vi "pathplan_vertices_send - 副本 (2).vi"(1 "vertices":dbl[][](array[numeric]), 2 "distance_all":dbl, 3 "angle_all":dbl[](array[numeric]), 4 "speed_max":dbl, 5 "写入串口":refnum<visa-resource-name>) -> (20 "路径规划数据写入缓冲区":string)   [LabVIEW 2016]
uses:
  <vilib>/imath/engines/lvmath2/RunTimeEngine/NodeEndStatement/NIMS_NodeEndStatement_Output.vi
  <instcachedir>/0/NIMS_NodeEndStatement_Output_53EC0D466D134D7ABD903AC30B43404B.lvgen/NIMS_NodeEndStatement_Output_53EC0D466D134D7ABD903AC30B43404B_011.vi
  <instcachedir>/0/NIMS_NodeEndStatement_Output_53EC0D466D134D7ABD903AC30B43404B.lvgen/NIMS_NodeEndStatement_Output_53EC0D466D134D7ABD903AC30B43404B_015.vi
  <vilib>/imath/engines/lvmath2/RunTimeEngine/ErrorHandling/NIMS_Finalize Error.vi
  <vilib>/imath/engines/lvmath2/RunTimeEngine/IndexRead/NIMS M($,S).vi
  <instcachedir>/0/NIMS M($,S)_3E5749BBB62E49528D4765A77F1F6D98.lvgen/NIMS M($,S)_3E5749BBB62E49528D4765A77F1F6D98_000.vi
  <vilib>/imath/engines/lvmath2/RunTimeEngine/ArithmeticOperatorToken/NIMS_ArithmeticOperator_minus.vi
  <instcachedir>/0/NIMS_ArithmeticOperator_minus_E3B65B1D26A44BB184AFDC5B3F458E3D.lvgen/NIMS_ArithmeticOperator_minus_E3B65B1D26A44BB184AFDC5B3F458E3D_003.vi
  <vilib>/imath/engines/lvmath2/RunTimeEngine/BuiltInFunctions/norm/NIMS_norm(GV,DBL).vi
  <instcachedir>/0/NIMS_norm(GV,DBL)_1268AFF3C646412B8C6EA3CE75D09042.lvgen/NIMS_norm(GV,DBL)_1268AFF3C646412B8C6EA3CE75D09042_000.vi
  <vilib>/imath/engines/lvmath2/RunTimeEngine/ErrorHandling/NIMS_Create Error From Enums.vi
  <vilib>/imath/engines/lvmath2/RunTimeEngine/BuiltInFunctions/length/NIMS_length(GM).vi
  <instcachedir>/0/NIMS_length(GM)_47CEC356FCE0482D9BA47DC61C99F2C7.lvgen/NIMS_length(GM)_47CEC356FCE0482D9BA47DC61C99F2C7_000.vi
  <vilib>/imath/engines/lvmath2/RunTimeEngine/RowToken/NIMS_RowToken_M_CV.vi
  <instcachedir>/0/NIMS_RowToken_M_CV_FA79F1D1D17D44459F3ED8E09EE8B625.lvgen/NIMS_RowToken_M_CV_FA79F1D1D17D44459F3ED8E09EE8B625_000.vi
  <vilib>/imathl/engines/lvmath/Functions/Error Handling/Create Error.vi
  <vilib>/imath/engines/lvmath2/RunTimeEngine/IndexRead/NIMS M($,R2).vi
  <instcachedir>/0/NIMS M($,R2)_D9380E19261A4ADFB2D364AF6959C6EF.lvgen/NIMS M($,R2)_D9380E19261A4ADFB2D364AF6959C6EF_001.vi
  <vilib>/imath/engines/lvmath2/RunTimeEngine/BuiltInFunctions/size/NIMS_I32=size(GM,I32).vi
  <instcachedir>/0/NIMS_I32=size(GM,I32)_122058B1B3294FAEA5DC209B92B394E4.lvgen/NIMS_I32=size(GM,I32)_122058B1B3294FAEA5DC209B92B394E4_004.vi
  <vilib>/imath/engines/lvmath2/RunTimeEngine/RangeToken/NIMS_Range_R2 - Integer.vi
  <instcachedir>/0/NIMS_Range_R2 - Integer_89B873E74E6E489885E44F751DD9C6BF.lvgen/NIMS_Range_R2 - Integer_89B873E74E6E489885E44F751DD9C6BF_000.vi
  <vilib>/imath/engines/lvmath2/RunTimeEngine/CommandStatement/MC_CommandStatement_break.vi
  <vilib>/imath/engines/lvmath2/RunTimeEngine/VariableToken/NIMS_VariableToken_CondDefined.vi
  <instcachedir>/0/NIMS_VariableToken_CondDefined_06E9DA95BD4D46A6BA55EC651A891960.lvgen/NIMS_VariableToken_CondDefined_06E9DA95BD4D46A6BA55EC651A891960_009.vi
  <vilib>/imath/engines/lvmath/Functions/Error Handling/MergeErrorsWrapper.vi
  <instcachedir>/0/NIMS_NodeEndStatement_Output_53EC0D466D134D7ABD903AC30B43404B.lvgen/NIMS_NodeEndStatement_Output_53EC0D466D134D7ABD903AC30B43404B_010.vi
  <instcachedir>/0/NIMS_NodeEndStatement_Output_53EC0D466D134D7ABD903AC30B43404B.lvgen/NIMS_NodeEndStatement_Output_53EC0D466D134D7ABD903AC30B43404B_005.vi
  <vilib>/imath/engines/lvmath2/RunTimeEngine/BuiltInFunctions/length/NIMS_length(GV).vi
  <instcachedir>/0/NIMS_length(GV)_08A3D13377FD4E4B96F5795FBF3698FA.lvgen/NIMS_length(GV)_08A3D13377FD4E4B96F5795FBF3698FA_000.vi
  <vilib>/imath/engines/lvmath2/RunTimeEngine/IndexRead/NIMS M(S,S).vi
  <instcachedir>/0/NIMS M(S,S)_AC51E74150A542F7991B9634C66F3096.lvgen/NIMS M(S,S)_AC51E74150A542F7991B9634C66F3096_000.vi
  <vilib>/imath/engines/lvmath2/RunTimeEngine/BuiltInFunctions/dot/NIMS_dot(GV,GV).vi
  <instcachedir>/0/NIMS_dot(GV,GV)_B9FAA411F4494E9B94D442721014A3FA.lvgen/NIMS_dot(GV,GV)_B9FAA411F4494E9B94D442721014A3FA_000.vi
  <vilib>/imath/engines/lvmath2/RunTimeEngine/IndexRead/NIMS V(S).vi
  <instcachedir>/0/NIMS V(S)_0488751826AF41519A22953C041130DC.lvgen/NIMS V(S)_0488751826AF41519A22953C041130DC_000.vi
  <instcachedir>/0/NIMS_NodeEndStatement_Output_53EC0D466D134D7ABD903AC30B43404B.lvgen/NIMS_NodeEndStatement_Output_53EC0D466D134D7ABD903AC30B43404B_009.vi
panel:
  in  "y":dbl
  in  "x":dbl
  in  "angle_z":sgl
  out "vertices_set":i32[][](array[numeric])
  out "angle_send":dbl[](array[numeric])
  out "vertices_send":dbl[](array[numeric])
  out "speed_send":dbl[](array[numeric])
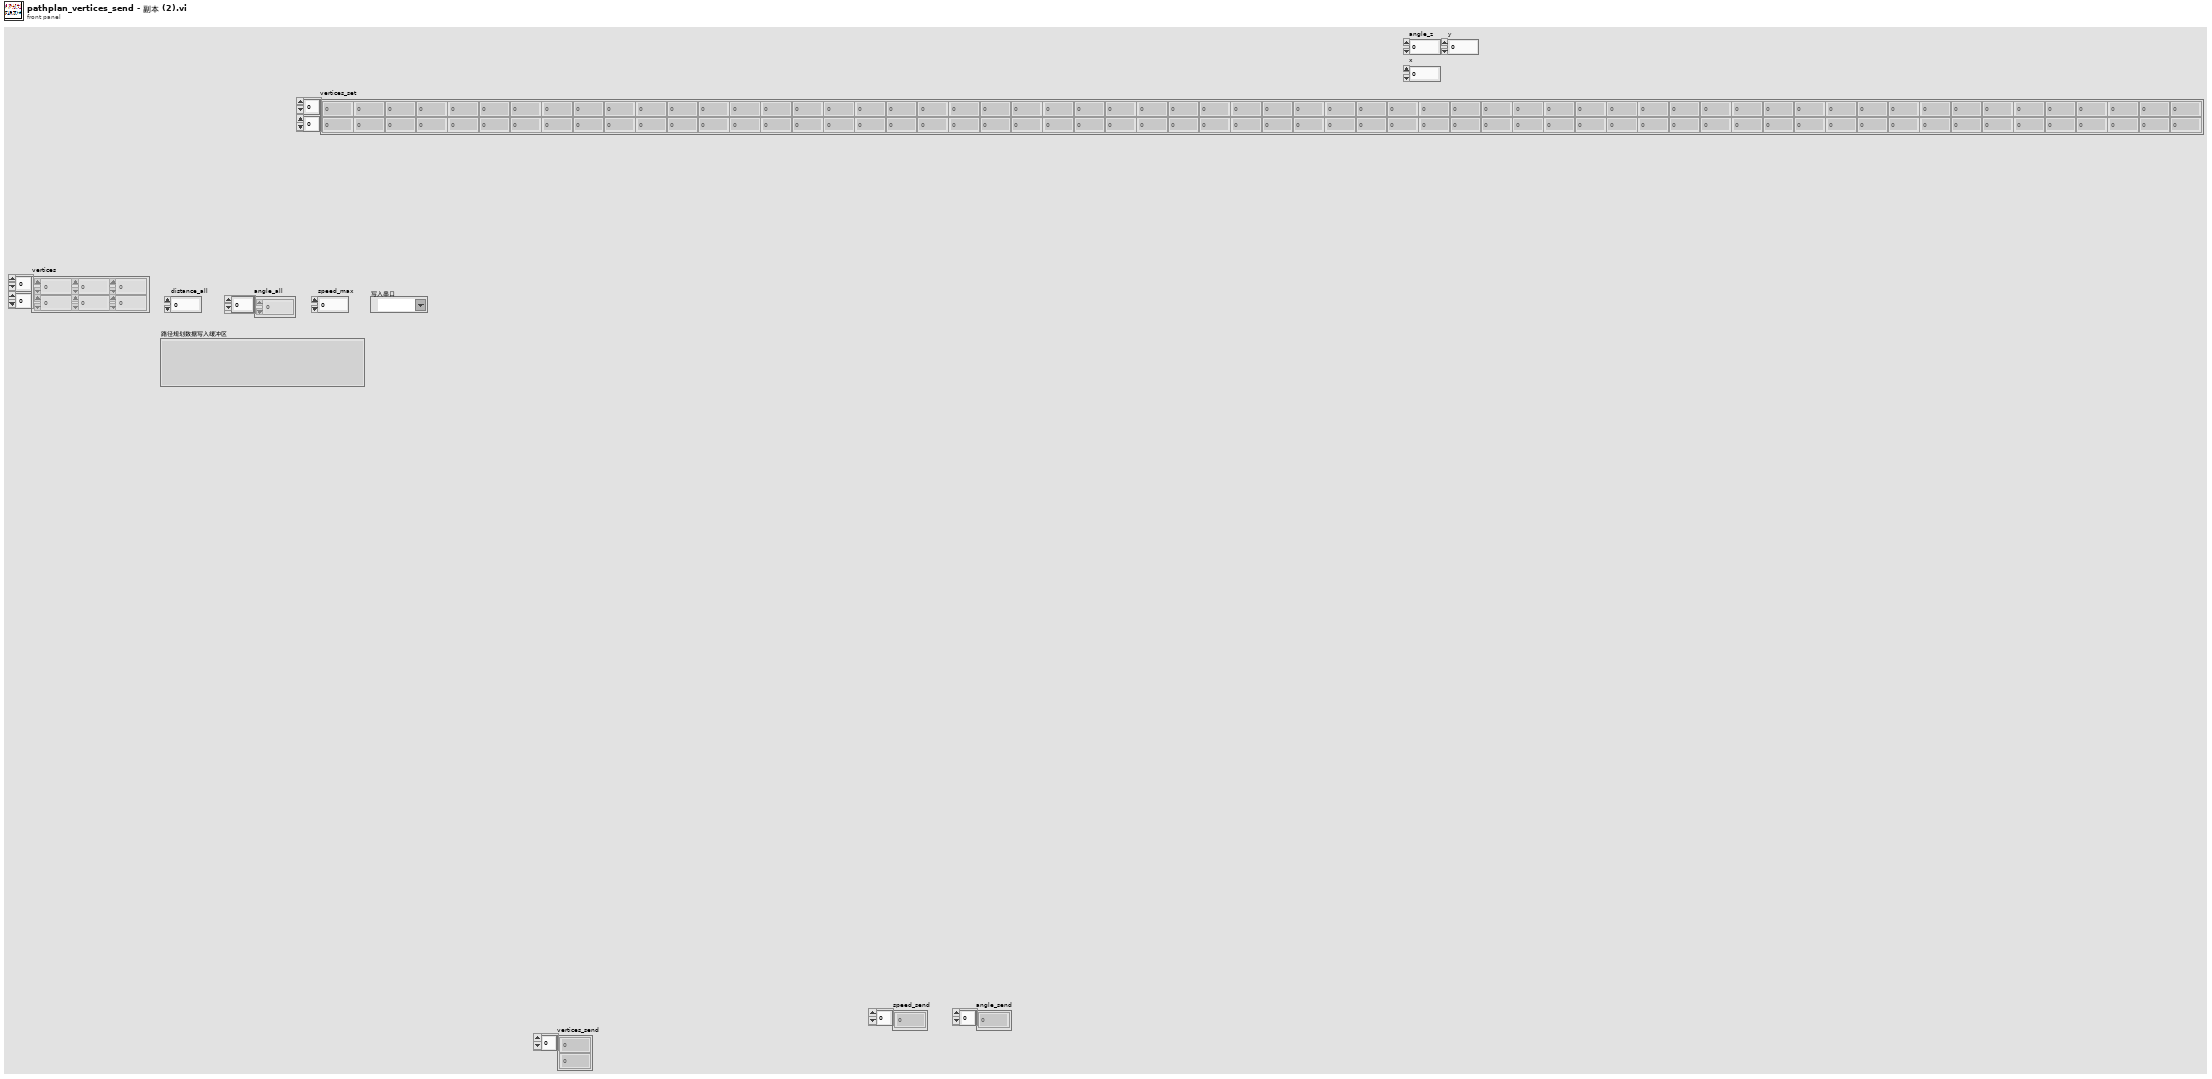
[diagram p1: front panel]
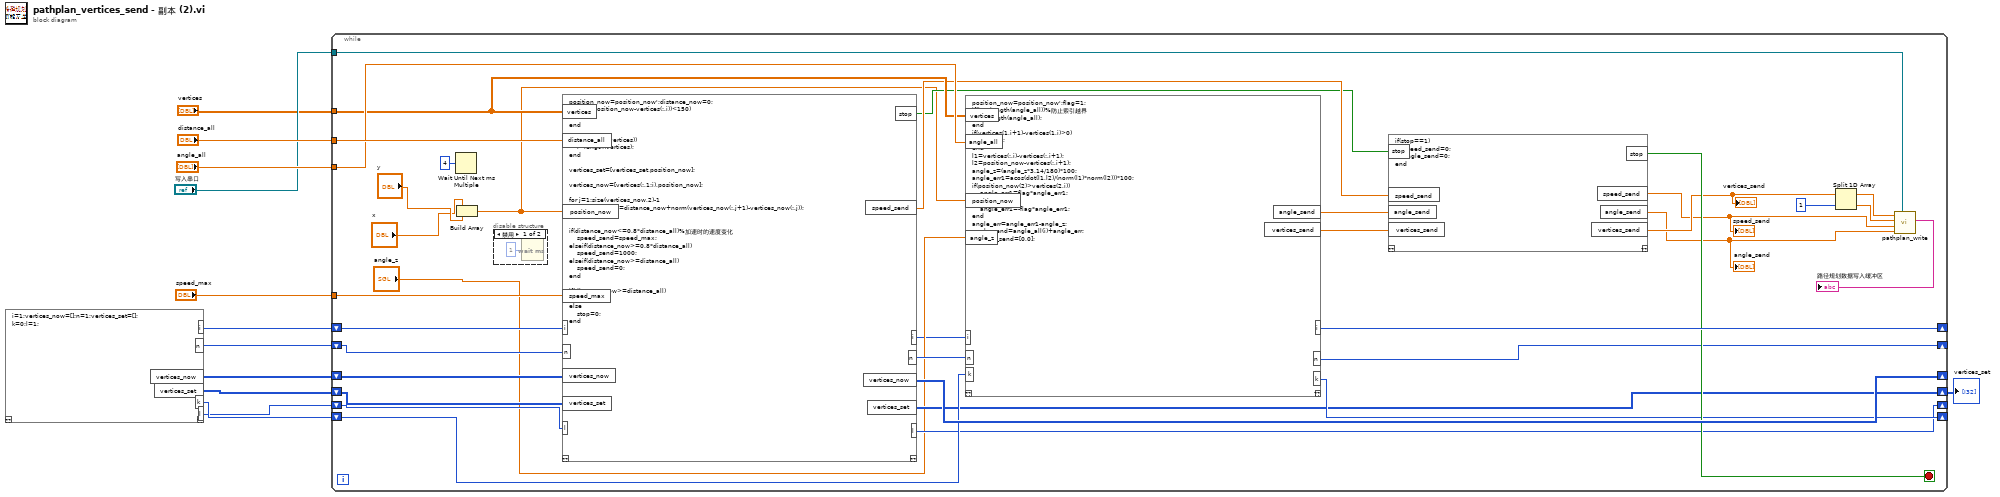
[diagram p0: block diagram]
diagram:
  n1 = mathscript code="i=1;vertices_now=[];n=1;vertices_set=[];\nk=0;l=1;"() -> ("i"=w10:i32, "vertices_now"=w8:i32[][], "n"=w5:i32, "vertices_set"=w3:i32[][], "k"=w4:i32, "l"=w2:i32)  [unwired: 1 in, 1 out]
  n2 = while {
    tunnel: "vertices" -> [w46]
    tunnel: "distance_all" -> [w48]
    tunnel: "angle_all" -> [w47]
    shift-right: [w45] -> _
    shift-left: w10 -> [w44]
    tunnel: "speed_max" -> [w43]
    shift-right: [w42] -> _
    shift-left: w8 -> [w28]
    tunnel: "写入串口" -> [w30]
    shift-right: [w25] -> _
    shift-left: w5 -> [w27]
    shift-right: [w23] -> _
    shift-left: w4 -> [w24]
    shift-right: [w18] -> w1
    shift-left: w3 -> [w21]
    shift-right: [w19] -> _
    shift-left: w2 -> [w20]
    stop <- w34 stop-if-true
    n3 = Wait Until Next ms Multiple(millisecond multiple=u32 4 ("毫秒倍数")) -> ()  [unwired: 1 out]
    n4 = Build Array("x", "y") -> (w22:dbl[])
    n5 = disable-structure shown="禁用" {
      frame Disabled {
        n6 = Wait (ms)(milliseconds to wait=u32 1 ("等待时间（毫秒）")) -> ()  [unwired: 1 out]
      }
      frame Enabled {
      }
    }
    n7 = mathscript code="position_now=position_now';distance_now=0;\nif(norm(position_now-vertices(:,i))<150)\n    i=i+1;\nend\n\nif(i>=length(vertices))\n    i=length(vertices);\nend\n\nvertices_set=[vertices_set,position_now];\n\nvertices_now=[vertices(:,1:i),position_now];\n\nfor j=1:size(vertices_now,2)-1\n    distance_now=distance_now+norm(vertices_now(:,j+1)-vertices_now(:,j));\nend\n\nif(distance_now<=0.8*distance_all)%加速时的速度变化\n    speed_send=speed_max;\nelseif(distance_now>=0.8*distance_all)\n    speed_send=1000;\nelseif(distance_now>=distance_all)\n    speed_send=0;\nend\n\nif(distance_now>=distance_all)\n    stop=0;\nelse\n    stop=0;\nend"("position_now"=w22, "vertices"=w46, "distance_all"=w48, "i"=w44, "speed_max"=w43, "vertices_now"=w28, "n"=w27, "vertices_set"=w21, "l"=w20) -> ("vertices_now"=w42:i32[][], "speed_send"=w37:dbl[], "stop"=w35:bool, "n"=w26:i32, "vertices_set"=w18:i32[][], "l"=w19:i32, "i"=w14:i32)  [unwired: 1 in, 1 out]
    n8 = mathscript code="position_now=position_now';flag=1;\nif(i>=length(angle_all))%防止索引越界\n    i=length(angle_all);\nend\nif(vertices(1,i+1)-vertices(1,i)>0)\n    flag=-1;\nend\nl1=vertices(:,i)-vertices(:,i+1);\nl2=position_now-vertices(:,i+1);\nangle_z=(angle_z*3.14/180)*100;\nangle_err1=acos(dot(l1,l2)/(norm(l1)*norm(l2)))*100;\nif(position_now(2)>vertices(2,i))\n    angle_err1=flag*angle_err1;\nelse\n    angle_err1=-flag*angle_err1;\nend\nangle_err=angle_err1-angle_z;\nangle_send=angle_all(i)+angle_err;\nvertices_send=[0,0];"("angle_all"=w47, "vertices"=w46, "position_now"=w22, "angle_z"="angle_z", "i"=w14, "n"=w26, "k"=w24) -> ("i"=w45:i32, "angle_send"=w38:cdb, "vertices_send"=w36:dbl[], "n"=w25:i32, "k"=w23:i32)  [unwired: 1 in, 1 out]
    n9 = mathscript code="if(stop==1)\n    speed_send=0;\n    angle_send=0;\nend"("speed_send"=w37, "angle_send"=w38, "vertices_send"=w36, "stop"=w35) -> ("stop"=w34:bool, "angle_send"=w31:dbl[], "speed_send"=w32:dbl[], "vertices_send"=w33:dbl[])  [unwired: 1 in, 1 out]
    "speed_send" <- w32
    "vertices_send" <- w33
    "angle_send" <- w31
    n10 = Split 1D Array(array=w33, index=1 ("索引")) -> (first subarray=w40:dbl[], second subarray=w39:dbl[])
    n11 = call "pathplan_write.vi"("VISA资源名称"=w30, "angle"=w31, "v"=w32, "y"=w39, "angle_err"=w40) -> ("路径规划数据写入缓冲区"=→"路径规划数据写入缓冲区":string)  [unwired: 6 in]
  }
  "vertices_set" <- w1
